vi "Main.vi"() -> ()   [LabVIEW 2022 SP3]
uses:
  TDs/FileProps.ctl
  TDs/PropToFilter.ctl
panel:
  out "Files":T1[](array[typedef])
  in  "Change filtered files":bool
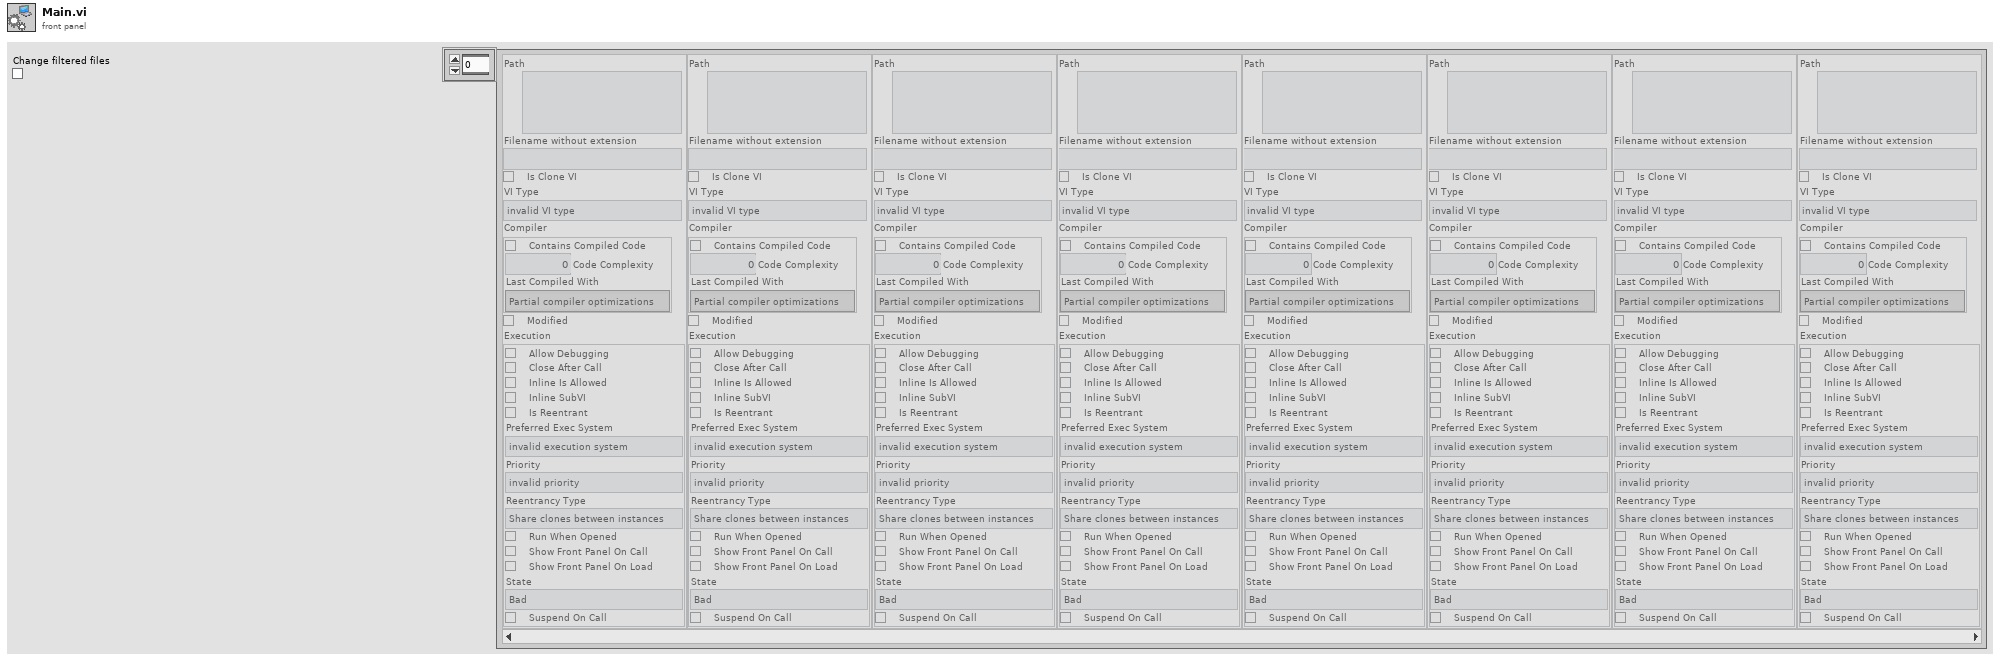
[diagram p1: front panel]
types:
  T1 = typedef "FileProps.ctl" = cluster{"Path":path, "Filename without extension":string, "Is Clone VI":bool, "VI Type":enum32{"invalid VI type", "Standard VI", "Control VI", "Global VI", "Polymorphic VI", "Configuration VI", "SubSystem", "Facade VI", "Method VI", "Statechart Diagram VI"}, "Compiler":cluster{"Contains Compiled Code":bool, "Code Complexity":sgl, "Last Compiled With":enum16{"Partial compiler optimizations", "Full compiler optimizations"}}, "Modified":bool, "Execution":cluster{"Allow Debugging":bool, "Close After Call":bool, "Inline Is Allowed":bool, "Inline SubVI":bool, "Is Reentrant":bool, "Preferred Exec System":enum32{"invalid execution system", "user interface", "standard", "instrument i/o", "data acquisition", "other 1", "other 2", "same as caller"}, "Priority":enum32{"invalid priority", "background priority", "normal priority", "above normal priority", "high priority", "time critical priority", "subroutine"}, "Reentrancy Type":enum16{"Share clones between instances", "Preallocate clone for each instance"}, "Run When Opened":bool, "Show Front Panel On Call":bool, "Show Front Panel On Load":bool, "State":enum32{"Bad", "Idle", "Run top level", "Running"}, "Suspend On Call":bool}}
  T2 = typedef "PropToFilter.ctl" = enum16{"None", "Prealloc Clones", "Separated Compiled Code", "Not Sep Compiled Code", "Modified"}
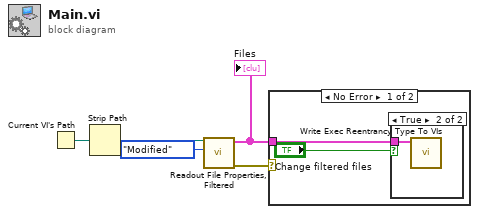
[diagram p0: block diagram]
diagram:
  n1 = Current VI's Path() -> (path=w4:path)
  n2 = Strip Path(path=w4) -> (stripped path=w1:path)  [unwired: 1 out]
  n3 = call "Readout File Properties, Filtered.vi"("Filter Type"=PropToFilter."Modified", "Selected Folder"=w1) -> ("error IO"=w3:errorcluster, "Files"=w5:T1[])  [unwired: 8 in]
  "Files" <- w5
  n4 = case shown="No Error" w3 {
    tunnel: w5 -> [w7 _]
    frame No Error {
      n5 = case shown="True" "Change filtered files" {
        tunnel: w7 -> [_ w8]
        frame False {
        }
        frame True {
          n6 = call "Write Exec Reentrancy Type To VIs.vi"("Array"=w8) -> ()  [unwired: 10 in, 1 out]
        }
      }
    }
    frame Error {
    }
  }
